vi "Double Preference.vi"(0 "key":string, 1 "section":string, 2 "Operation":enum16{"Load", "Save"}(ring)=enum."Save", 3 "refnum in":T1, 9 "default value":dbl) -> (12 "section out":string, 13 "Operation out":enum16{"Load", "Save"}(ring)=enum."Save", 14 "refnum out":T1)   [LabVIEW 2013]
uses:
  <vilib>/Utility/config.llb/Config Data RefNum.ctl
  <vilib>/Utility/config.llb/Read Key (Double).vi
  <vilib>/Utility/config.llb/Write Key (Double).vi
  <vilib>/Utility/config.llb/NI_LVConfig.lvlib
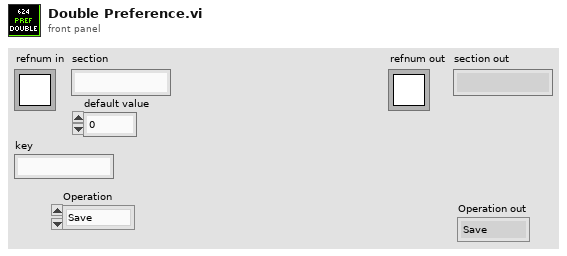
[diagram p1: front panel]
types:
  T1 = typedef "NI_LVConfig.lvlib/Config Data RefNum.ctl" = refnum<k1>
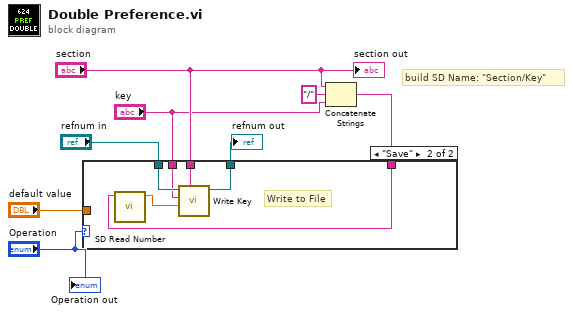
[diagram p0: block diagram]
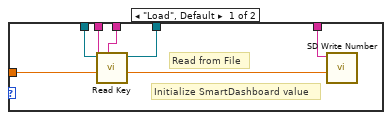
[diagram p2: hidden frame]
diagram:
  # "build SD Name: \"Section/Key\""
  n1 = Concatenate Strings("section", "/" ("string"), "key") -> (w2:string)
  n2 = case shown="\"Save\"" "Operation" {
    tunnel: "refnum in" -> [w15 w21]
    tunnel: [w14 w20] -> w7
    tunnel: "default value" -> [w13 _]
    tunnel: "section" -> [w12 w18]
    tunnel: "key" -> [w11 w19]
    tunnel: w2 -> [w10 w17]
    frame "Load", Default {
      # "Initialize SmartDashboard value"
      # "Read from File"
      n3 = call-poly <vilib>:"Read Key.vi"("section"=w12, "default value"=w13, "key"=w11, "refnum"=w15) -> ("value"=w9:dbl, "refnum out"=w14:T1)  [unwired: 4 in, 2 out]
      n4 = call <vilib>:"SD Write Number.vi"("Numeric"=w9, "Name"=w10) -> ()  [unwired: 8 in, 2 out]
    }
    frame "Save" {
      # "Write to File"
      n5 = call <vilib>:"SD Read Number.vi"("Name"=w17) -> ("Numeric"=w16:dbl)  [unwired: 8 in, 2 out]
      n6 = call-poly <vilib>:"Write Key.vi"("section"=w18, "value"=w16, "key"=w19, "refnum"=w21) -> ("refnum out"=w20:T1)  [unwired: 5 in, 2 out]
    }
  }
  "refnum out" <- w7
  "section out" <- "section"
  "Operation out" <- "Operation"
